vi "New Credit.vi"(8 "error in (no error)":errorcluster, 10 "Nw Credit":dbl, 11 "Actor_USD in":refnum<class "Actor_USD.lvclass">) -> (0 "error out":errorcluster, 3 "Actor_USD out":refnum<class "Actor_USD.lvclass">)   [LabVIEW 2019, in "Actor_USD.lvlib" / "Actor_USD.lvclass"]
uses:
  Actor_USD.lvclass
  Actor_USD.lvclass/Actor_USD.ctl
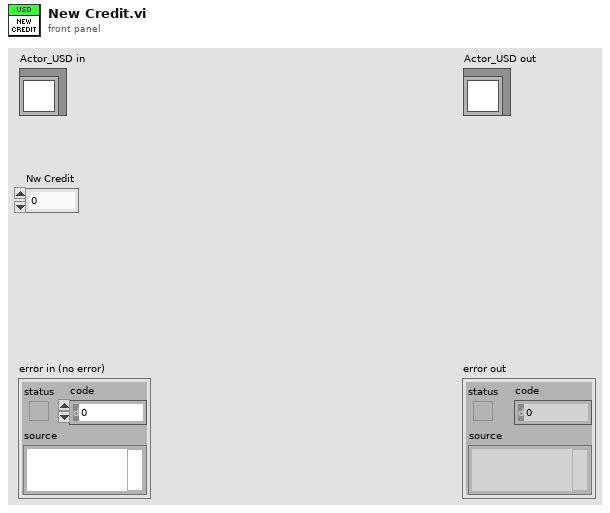
[diagram p1: front panel]
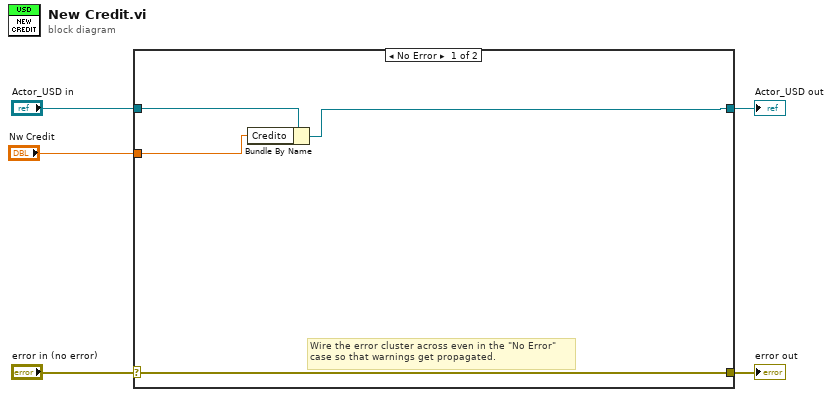
[diagram p0: block diagram]
diagram:
  n1 = case shown="No Error" "error in (no error)" {
    selector: "error in (no error)" -> [w9 w11]
    tunnel: [w9 w11] -> w4
    tunnel: [w7 w10] -> w2
    tunnel: "Actor_USD in" -> [w8 w10]
    tunnel: "Nw Credit" -> [w6 _]
    frame No Error {
      # "Wire the error cluster across even in the \"No Error\"\ncase so that warnings get propagated."
      n2 = Bundle By Name(cluster=w8, "Credito"=w6) -> (w7:refnum<class "Actor_USD.lvclass">)
    }
    frame Error {
    }
  }
  "error out" <- w4
  "Actor_USD out" <- w2
